vi "CreateGigEHandle.vi"(7 "error in (no error)":errorcluster caption="错误输入（无错误）", 9 "GigEDevice":T1) -> (0 "error out":errorcluster caption="错误输出", 2 "handle":u64, 3 "function return":i32)   [LabVIEW 2015, in "MvCameraControl.lvlib"]
doc: "MV_LV_API int __stdcall CreateHandle(void ** handle, const MV_CC_DEVICE_INFO* pstDevInfo);"
uses:
  MvCameraControl.lvlib
  MvCameraPatch.dll
types:
  T1 = cluster{"nMajorVer":u16, "nMinorVer":u16, "nMacAddrHigh":u32, "nMacAddrLow":u32, "nTLayerType":u32, "nReserved0":u32, "nReserved1":u32, "nReserved2":u32, "nReserved3":u32, "nIpCfgOption":u32, "nIpCfgCurrent":u32, "nCurrentIp":u32, "nCurrentSubNetMask":u32, "nDefaultGateWay":u32, "chManualfacturerName":string, "chModelName":string, "chDeviceVersion":string, "chManufacturerSpecificInfo":string, "chSerialNumber":string, "chUserDefinedName":string, "nNetExport":u32, "nRes0":u32, "nRes1":u32, "nRes2":u32, "nRes3":u32}
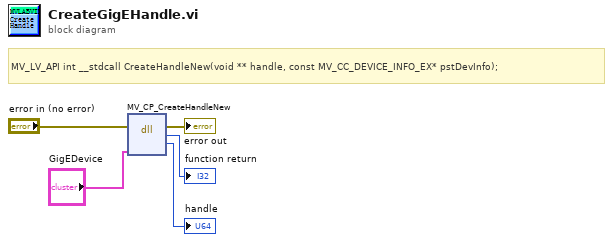
[diagram p0: block diagram]
diagram:
  # "MV_LV_API int __stdcall CreateHandleNew(void ** handle, const MV_CC_DEVICE_INFO_EX* pstDevInfo);"
  n1 = dll-call lib="MvCameraPatch.dll" fn="MV_CP_CreateHandleNew"(error in="error in (no error)", "pstDevInfo"="GigEDevice") -> (error out=→"error out":errorcluster, "返回类型"=→"function return":i32, "handle"=→"handle":u64)  [unwired: 4 in, 1 out]
